vi "winchcontrol2014_preT-Tide.vi"() -> ()   [LabVIEW 2014]
uses:
  Instance           1 20Saved   winchcontrol .vi
  Instance           2 20Saved   winchcontrol .vi
  Instance           4 20Saved   winchcontrol .vi
  Instance           3 20Saved   winchcontrol .vi
  Instance           5 20Saved   winchcontrol .vi
  Instance           6 20Saved   winchcontrol .vi
panel:
  in  "Path of Image Capture":path=path "/OPG_Winch_MiniCoreDuo/Users/opg/Sites/FCTD_WINCH/LabView.png"
  in  "Screen Capture":bool
  out "Last update string":string="Updated: 10/29/12 6:37:41 PM"
  in  "Port":i32=4050
  in  "Red Lion IP Address":string="192.168.1.160"
  in  "Beep\non wait?":bool=TRUE
  in  "Drive by \nCTD Data":bool=TRUE
  out "isMaxPaySet":bool
  out "Old Max Payout":dbl=500.0
  in  "Maximum depth [m]":dbl=330.0 min=0.0 max=2000.0 step=1.0 format="%#_4f"
  out "Time @ max":timestamp=timestamp(3434357554.995505 s since 1904-01-01) format="%<%H:%M:%S>T"
  out "Max payout":dbl=26.1 format="%#_6f"
  out "Max depth":dbl format="%#_6f"
  in  "Go Up Now":bool
  in  "EMERGENCY\n      STOP":bool=TRUE caption="STOP!!!!!"
  in  "Final In Speed\n[turns/sec]":dbl=0.7 min=0.0 max=4.0 step=0.1 format="%_2f"
  in  "Slow depth\n[turns]":dbl=7.0 min=0.0 max=1500.0 step=1.0
  out "Final in Speed":dbl=0.7 min=0.0 max=4.0 step=0.1 format="%3_2g"
  out "Slow Depth":dbl=7.0 min=0.0 max=4.0 step=0.1
  out "Depth Derivative":dbl(graph)=0.09403073471738166
  out "CTD Com Miss Count":dbl
  out "Winch Com Miss Count":dbl=1.0
  out "Sax Status":u8[](array[numeric])=[1, 1, 0, 0, 5, 0, 1, 1, 0, 0]
  out "Pressure":dbl(graph)=1.818078
  out "i value":i32
  out "concatenated string":string="$OPGST,1,2,1243"
  out "CTD data":string="2615984408,1.818078,23.842880,5.097004"
  out "Depth":dbl(slide)=1.8080824462346528 min=0.0 max=1200.0 scale format="%#_4f"
  out "*(type *) &x":i32=38
  out "timestamp":u32=2615984408
  out "Temperature":dbl(graph)=23.84288
  out "Parameter String":string="$reqparmx:0019;0000$OPGWPM,10,16,+   6,+ 500, 4.2, 2.0,10000,10000,20000,40000,60000,60000,    0.70,    7,;"
  out "Status String":string="$OPGWST,3,1,+   1.8, 266.9,   0,- 0.01,   0.00,   0,   26307,;"
  out "Sax Status Code":dbl=26307.0 format="%#_8f"
  out "Motor Current":dbl
  out "Motor Payout":dbl=266.9
  out "Sheave Payout":dbl
  out "ATM90 Payout":dbl=1.8
  in  "CTD Data  IP Address":string="192.168.1.158"
  in  "Port":i32=2342
  out "bytes written":i32=62
  out "RL Status Received":bool=TRUE
  out "Acc Out":dbl=10000.0
  out "Acc In":dbl=10000.0
  out "Winch Action Status":T1(ring)=enum."HOMING"
  out "Winch Control Mode":T2(ring)=enum."AUTO"
  out "Decel Stop In":dbl=60000.0
  out "Decel Stop Out":dbl=60000.0
  out "Decel In":dbl=40000.0
  out "Decel Out":dbl=20000.0
  out "Wire In Speed":dbl=2.0
  out "Wire Out Speed":dbl=4.2
  out "Min Payout":dbl=6.0
  out "Max Payout":dbl=500.0
  out "I Limit Out":dbl=10.0
  out "I Limit In":dbl=16.0
  in  "Drop time [min.]":dbl=8.099999999999985 min=0.0 step=0.1 format="%.1f"
  out "output":string
  in  "Stop Now":bool
  in  "Wire In Speed\n[turns/sec]":dbl=2.0 min=0.0 max=5.0 step=0.1 format="%3_2f"
  in  "Decel in":dbl=40000.0
  in  "Decel out":dbl=20000.0
  in  "Stop decel in":dbl=60000.0
  in  "Stop decel out":dbl=60000.0
  in  "Accel  in":dbl=10000.0
  in  "Accel out":dbl=10000.0
  in  "Current limit out\n[Amps]":dbl=10.0 min=0.0 max=20.0 step=0.1 format="%_3f"
  in  "Current limit in\n[Amps]":dbl=16.0 min=0.0 max=18.0 format="%_3f"
  out "input 2":string="$reqparmx:0019;0000$OPGWPM,10,16,+   6,+ 500, 4.2, 2.0,10000,10000,20000,40000,60000,60000,    0.70,    7,;"
  out "Depth History":cluster{"Depth":dbl, "Value":dbl}(graph)={"Depth"=1.818078, "Value"=1.8}
  out "Payout":dbl(slide)=1.8 min=0.0 max=1200.0 step=200.0 scale format="%#1_3f"
  out "Velocity Now":dbl(knob)=-0.01 min=-5.0 max=5.0 step=1.0 scale=-5.0..5.0 scale format="%#_1f"
  in  "Maximum payout [turns]":dbl=500.0 min=0.0 max=1640.0 step=1.0 format="%#_4f"
  in  "Minimum payout [turns]":dbl=6.0 min=0.0 max=2000.0 step=1.0
  in  "Winch Auto Run":bool=TRUE
  out "Enabled":bool=TRUE
  in  "Wire Out Speed\n[turns/sec]":dbl=4.2 min=0.0 max=8.0 step=0.1 format="%_2f"
  out "Target\nDepth":dbl
  out "Conductivity":dbl(graph)=5.097004
  # "OPG  FAST  CTD"
  # "Winch Variable Status"
  # "Winch Variable Controls"
  # "FCTD DATA COMMUNICATION SETUP"
  # "RED LION CONTROL PANEL COM."
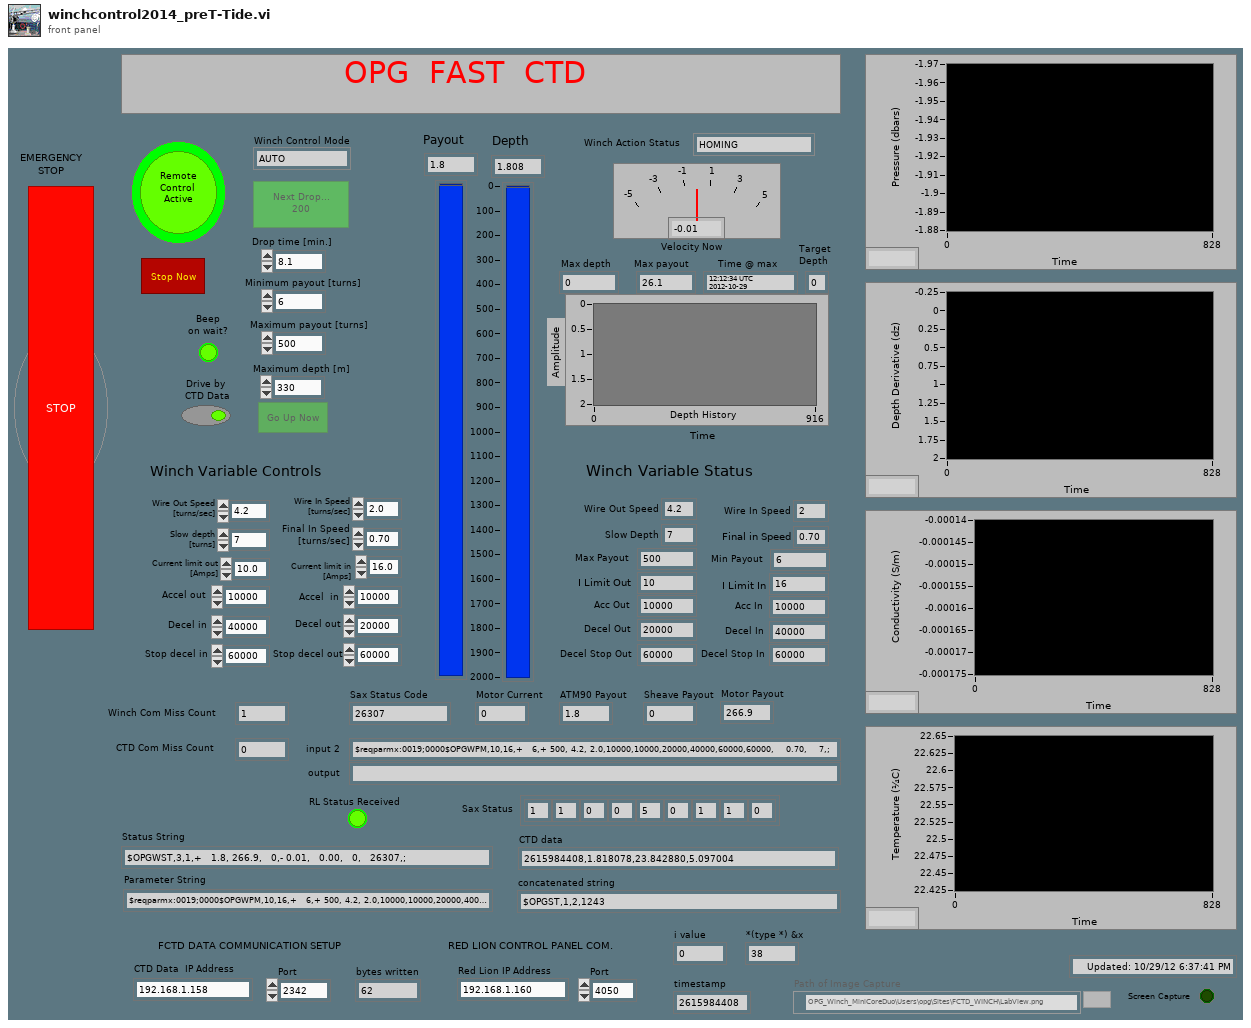
[diagram p1: front panel]
types:
  T1 = enum16{"START HOMING", "HOMING", "WAIT FOR TRIGGER", "START DROP", "GOING DOWN ?", "GOING UP"}
  T2 = enum16{"STOPPED", "MANUAL JOY", "MANUAL POT", "AUTO", "SEMIAUTO"}
  T3 = cluster{"Array[0]":dbl, "Array[1]":dbl, "Array[2]":dbl, "Array[3]":dbl, "Array[4]":dbl, "Array[5]":dbl, "Array[6]":dbl, "Array[7]":dbl, "Array[8]":dbl}
  T4 = cluster{"Array[0]":dbl, "Array[1]":dbl, "Array[2]":dbl, "Array[3]":dbl, "Array[4]":dbl, "Array[5]":dbl, "Array[6]":dbl, "Array[7]":dbl, "Array[8]":dbl, "Array[9]":dbl, "Array[10]":dbl, "Array[11]":dbl, "Array[12]":dbl, "Array[13]":dbl}
  T5 = typedef "imagedata.ctl" = cluster{"image type":i32, "image depth":i32, "image":u8[], "mask":u8[], "colors":u32[], "Rectangle":cluster{"left":i16, "top":i16, "right":i16, "bottom":i16}}
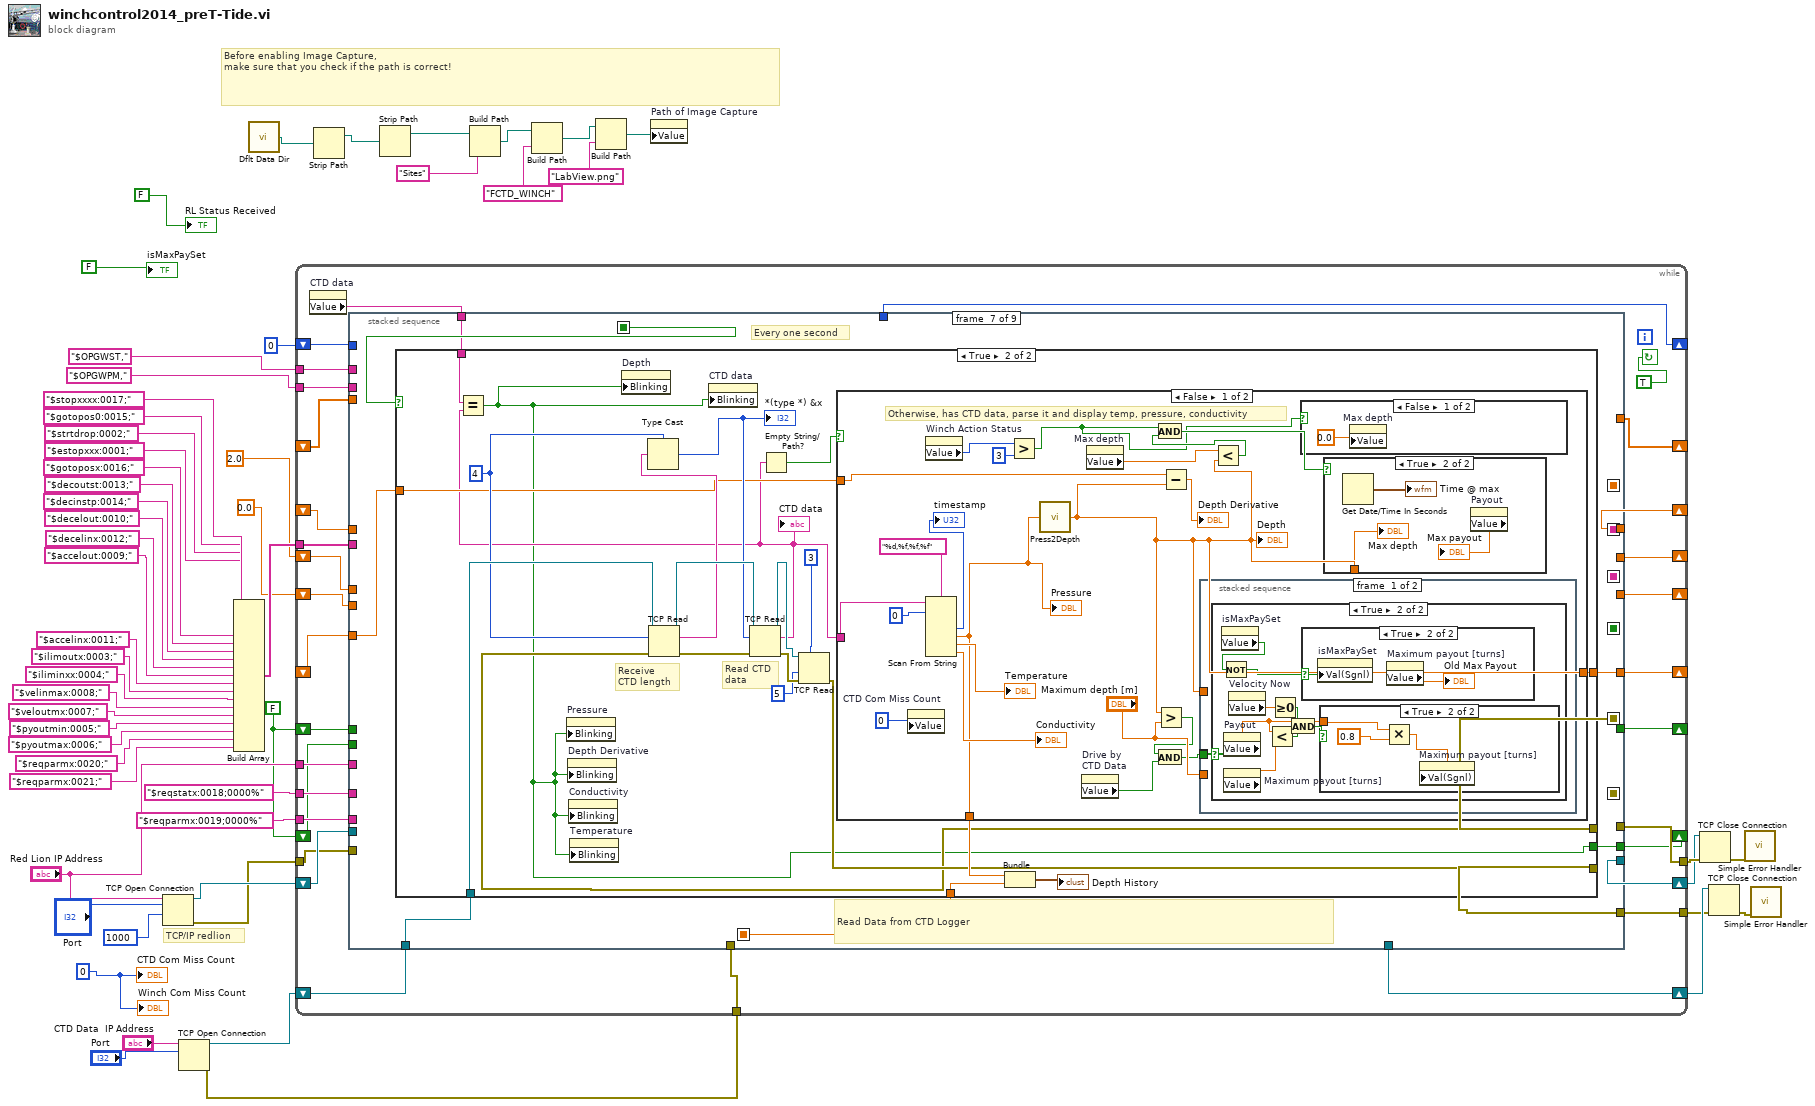
[diagram p0: block diagram]
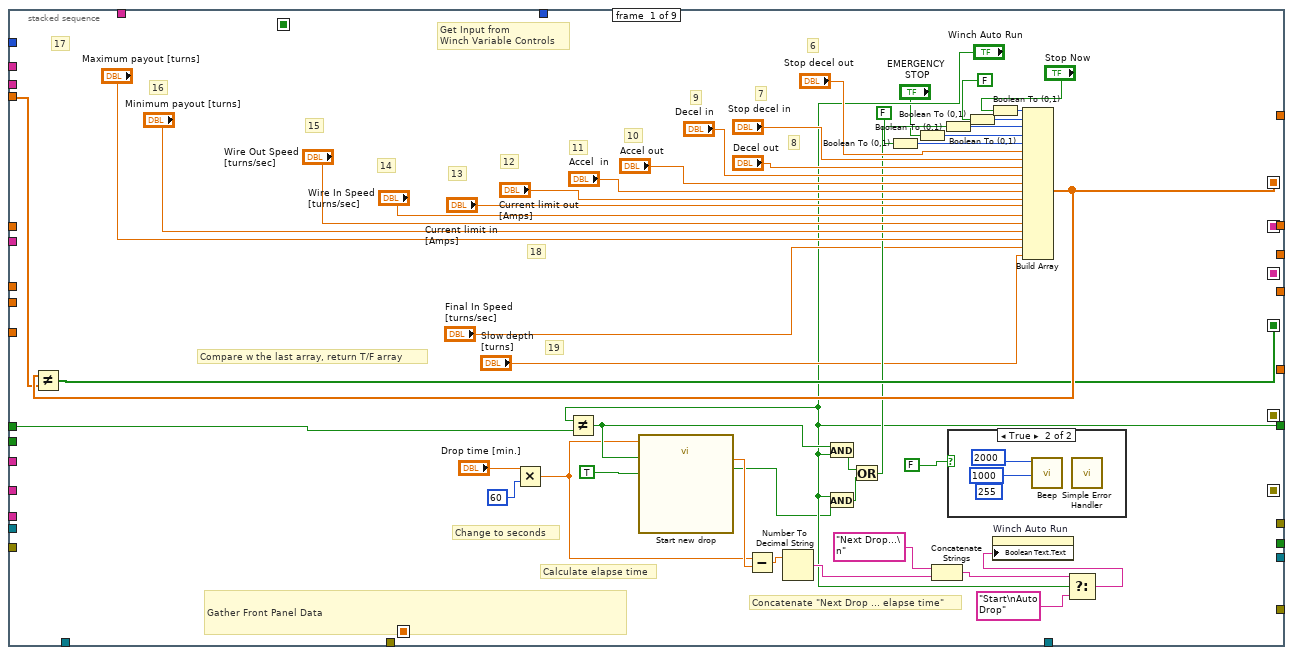
[diagram p2: hidden frame]
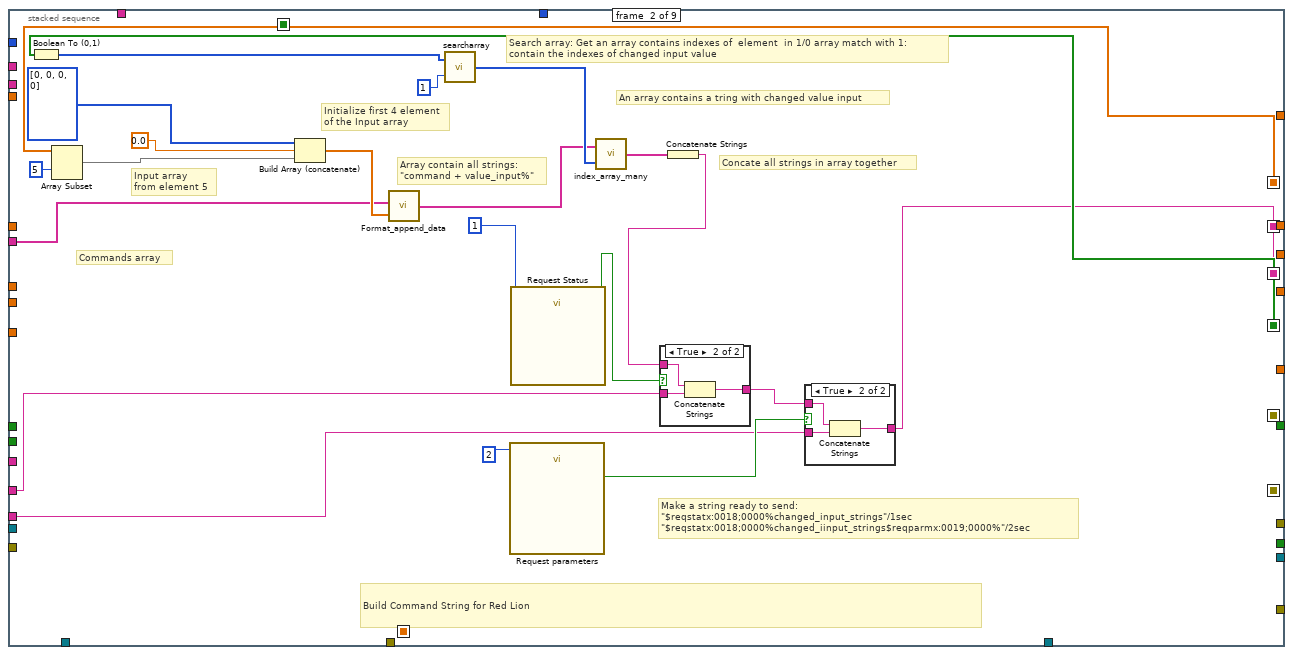
[diagram p4: hidden frame]
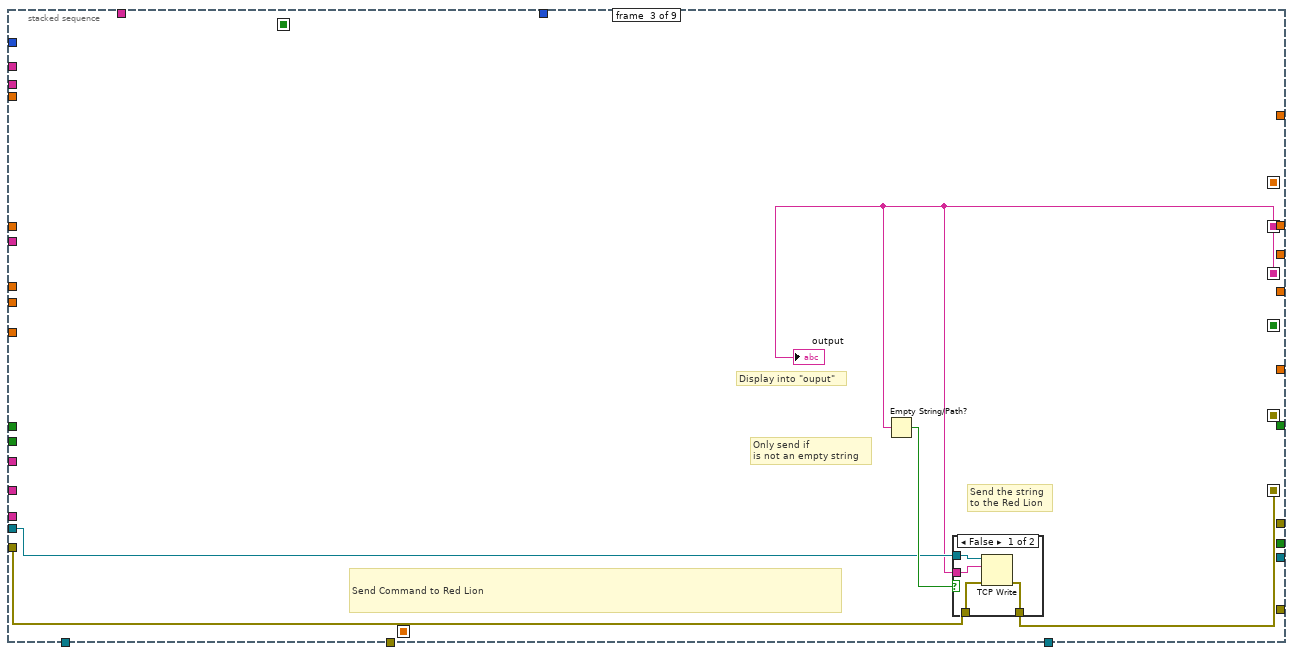
[diagram p7: hidden frame]
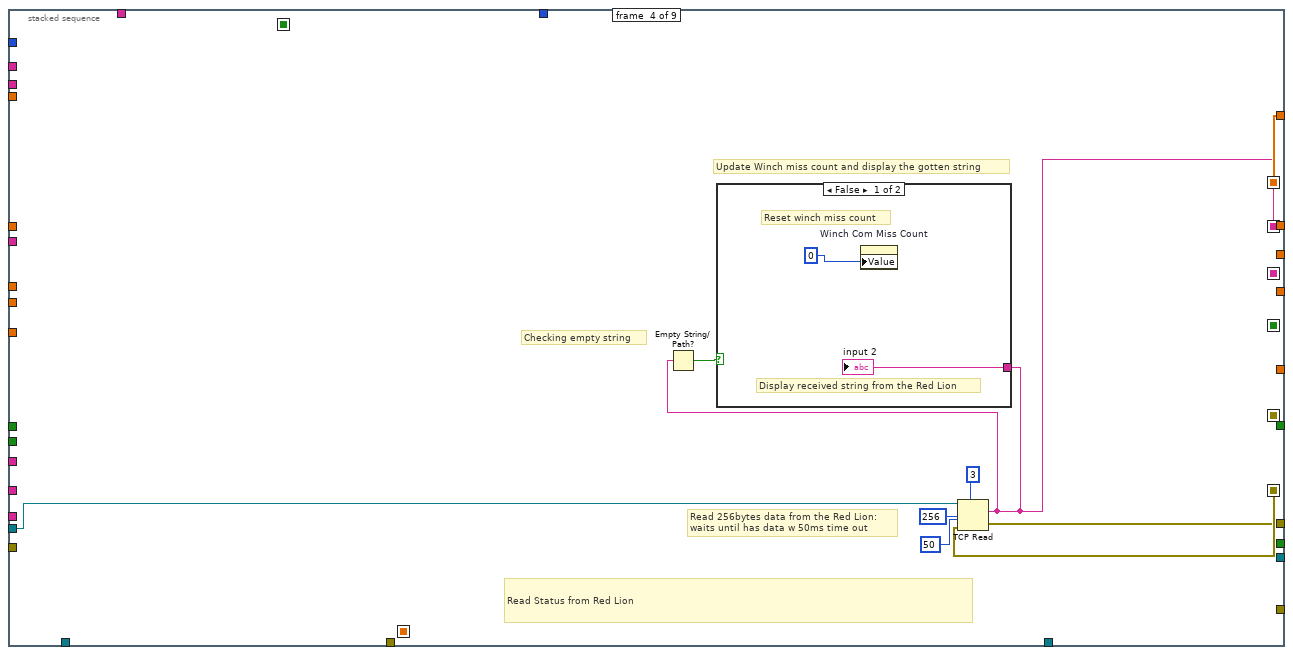
[diagram p9: hidden frame]
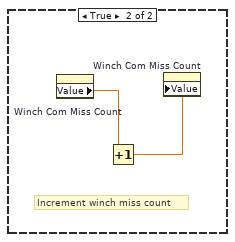
[diagram p10: hidden frame]
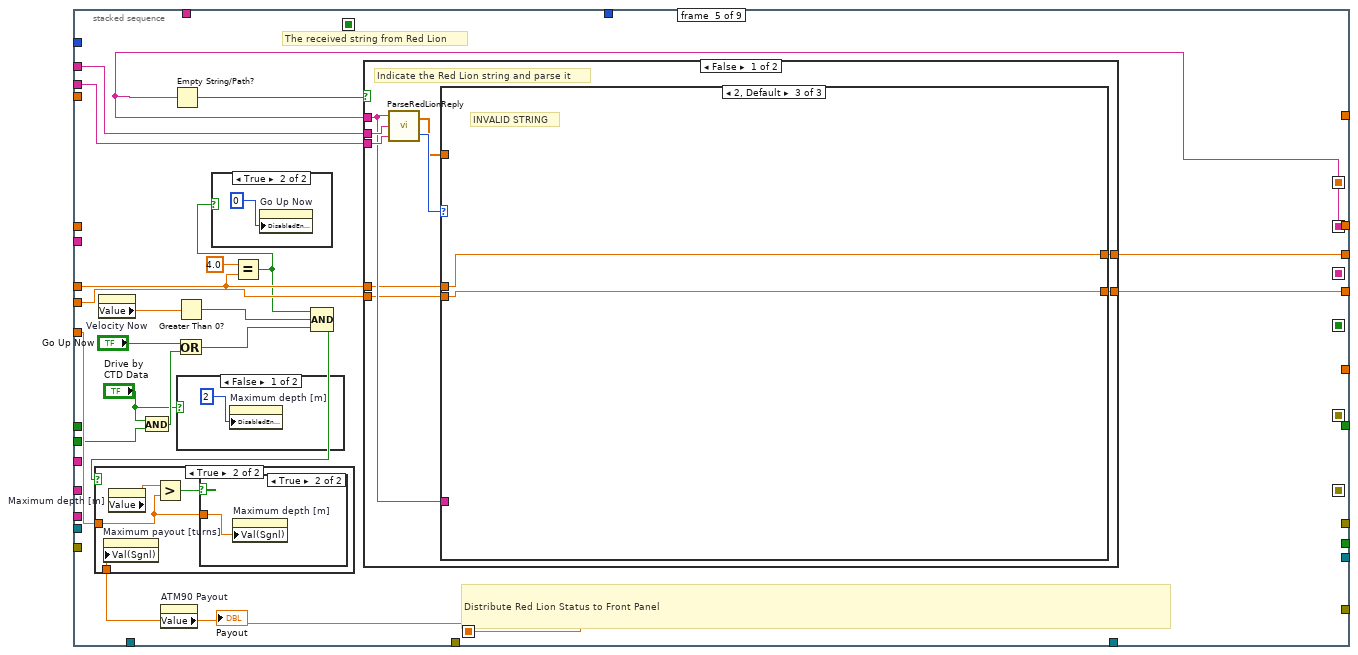
[diagram p11: hidden frame]
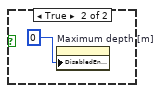
[diagram p12: hidden frame]
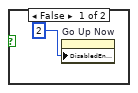
[diagram p13: hidden frame]
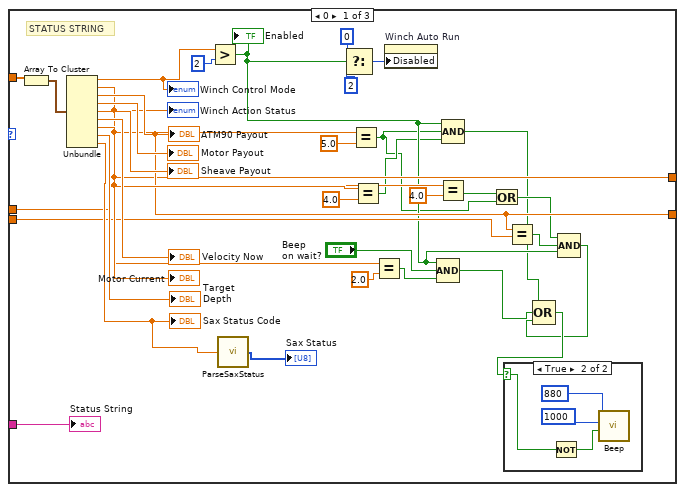
[diagram p16: hidden frame]
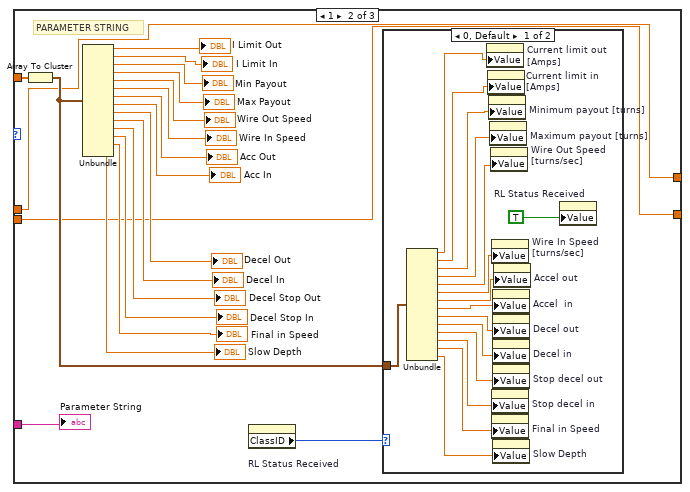
[diagram p18: hidden frame]
diagram:
  w12 = FALSE
  w19 = 0
  # "Before enabling Image Capture, \nmake sure that you check if the path is correct!"
  # "TCP/IP redlion"
  n1 = TCP Open Connection(address="Red Lion IP Address", remote port or service name="Port", timeout ms (60000)=1000) -> (connection ID=w54:refnum<k5>, error out=w52:errorcluster)  [unwired: 2 in]
  n2 = TCP Open Connection(address="CTD Data  IP Address", remote port or service name="Port") -> (connection ID=w28:refnum<k5>, error out=w26:errorcluster)  [unwired: 3 in]
  n3 = Build Array("$stopxxxx:0017;", "$gotopos0:0015;", "$strtdrop:0002;", "$estopxxx:0001;", "$gotoposx:0016;", "$decoutst:0013;", "$decinstp:0014;", "$decelout:0010;", "$decelinx:0012;", "$accelout:0009;", "$accelinx:0011;", "$ilimoutx:0003;", "$iliminxx:0004;", "$velinmax:0008;", "$veloutmx:0007;", "$pyoutmin:0005;", "$pyoutmax:0006;", "$reqparmx:0020;", "$reqparmx:0021;") -> (w50:string[])
  n4 = call <vilib>:"Dflt Data Dir.vi"() -> ("App:Default Data Directory"=w9:path)
  n5 = while {
    shift-right: [w87] -> _
    shift-left: _ -> [w85]
    tunnel: w52 -> [w82]
    tunnel: [w86] -> w51
    tunnel: w50 -> [w84]
    tunnel: "$reqstatx:0018;0000%" -> [w81]
    shift-right: [w80] -> _
    shift-left: w12 -> [w79]
    tunnel: w26 -> [w77]
    tunnel: [w76] -> w25
    tunnel: "$reqparmx:0019;0000%" -> [w75]
    shift-right: [w74] -> _
    shift-left: _ -> [w73]
    shift-right: [w72] -> _
    shift-left: 0 -> [w71]
    tunnel: "$OPGWST," -> [w70]
    tunnel: "$OPGWPM," -> [w69]
    shift-right: [w67] -> w18
    shift-left: w54 -> [w83]
    shift-right: [w66] -> w27
    shift-left: w28 -> [w78]
    shift-right: [w65] -> _
    shift-left: _ -> [w64]
    tunnel: "Red Lion IP Address" -> [w62]
    shift-right: [w61] -> _
    shift-left: w12 -> [w60]
    shift-right: [w59] -> _
    shift-left: 2.0 -> [w58]
    shift-right: [w57] -> _
    shift-left: 0.0 -> [w56]
    stop <- TRUE continue-if-true
    n6 = property on="CTD data" class="Str"() -> ("Value"=w63:string)  [unwired: 2 in, 2 out]
    n7 = stacked-sequence {
      seq-local: [w132 _ _ _ _ _ _ _ _] -> [_ w149 _ w183 _ _ _ _ _]
      seq-local: [_ w135 _ _ _ _ _ _ _] -> [_ _ w165 _ _ _ _ _ _]
      seq-local: [_ _ w166 _ _ _ _ _ _] -> [_ _ _ w178 _ _ _ _ _]
      seq-local: [w128 _ _ _ _ _ _ _ _] -> [_ w156 _ _ _ _ _ _ _]
      seq-local: [_ _ _ w176 _ _ _ _ _] -> [_ _ _ _ w205 _ _ _ _]
      seq-local: [_ _ _ _ _ w311 _ _ _] -> [_ _ _ _ _ _ w357 _ _]
      seq-local: [_ _ _ _ w203 _ _ _ _] -> [_ _ _ _ _ _ w355 _ _]
      seq-local: [_ _ _ _ _ w310 _ _ _] -> [_ _ _ _ _ _ w354 _ _]
      tunnel: w82 -> [_ _ w168 _ _ _ _ _ _]
      tunnel: w83 -> [_ _ w167 w179 _ _ _ w445 _]
      tunnel: [_ _ _ w183 _ _ _ _ _] -> w87
      tunnel: w84 -> [_ w147 _ _ _ _ _ _ _]
      tunnel: [_ _ _ w177 _ _ _ _ _] -> w86
      tunnel: w85 -> [w131 _ _ _ _ _ _ _ _]
      tunnel: w81 -> [_ w141 _ _ _ _ _ _ _]
      tunnel: ["Winch Auto Run" _ _ _ _ _ _ _ _] -> w80
      tunnel: w79 -> [w106 _ _ _ _ _ _ _ _]
      tunnel: w78 -> [_ _ _ _ _ w313 w358 w443 _]
      tunnel: w77 -> [_ _ _ _ _ w312 _ _ _]
      tunnel: [_ _ _ _ _ _ w356 _ _] -> w76
      tunnel: w75 -> [_ w136 _ _ _ _ _ _ _]
      tunnel: [_ _ _ _ _ w308 _ _ _] -> w74
      tunnel: w73 -> [_ _ _ _ _ w307 _ _ _]
      tunnel: w71 -> [_ _ _ _ _ w306 _ _ _]
      tunnel: [_ _ _ _ _ w305 _ _ _] -> w72
      tunnel: w70 -> [_ _ _ _ w207 _ _ _ _]
      tunnel: w69 -> [_ _ _ _ w206 _ _ _ _]
      tunnel: [_ _ _ _ _ _ _ w444 _] -> w67
      tunnel: [_ _ _ _ _ _ _ w442 _] -> w66
      tunnel: [_ _ _ _ _ _ w353 _ _] -> w65
      tunnel: w64 -> [_ _ _ _ w199 _ w352 _ _]
      tunnel: w63 -> [_ _ _ _ _ _ w351 _ _]
      tunnel: w62 -> [_ _ _ _ _ _ _ w441 _]
      tunnel: [_ _ _ _ _ _ w350 _ _] -> w61
      tunnel: w60 -> [_ _ _ _ w196 _ _ _ _]
      tunnel: [_ _ _ _ w193 _ _ _ _] -> w59
      tunnel: w58 -> [_ _ _ _ w189 _ _ _ _]
      tunnel: [_ _ _ _ w192 _ _ _ _] -> w57
      tunnel: w56 -> [_ _ _ _ w191 _ _ _ _]
      frame #0 {
        w129 = FALSE items=["OFF", "ON", "OFF", "ON"] ("Return to top")
        w115 = FALSE items=["OFF", "ON", "OFF", "ON"] ("Go to ...")
        # "19"
        # "18"
        # "17"
        # "16"
        # "15"
        # "14"
        # "13"
        # "12"
        # "11"
        # "10"
        # "9"
        # "8"
        # "7"
        # "6"
        # "Compare w the last array, return T/F array"
        # "Concatenate \"Next Drop ... elapse time\""
        # "Calculate elapse time"
        # "Change to seconds"
        # "Get Input from\nWinch Variable Controls"
        # "Gather Front Panel Data"
        n8 = Multiply(x="Drop time [min.]", y=60) -> (x*y=w100:dbl)
        n9 = Not Equal?(x="Winch Auto Run", y=w106) -> (x != y?=w105:bool)
        n10 = call "Start new drop"("Time Target (s)"=w100, "Reset"=w105, "Auto Reset"=TRUE) -> ("Elapsed Time (s)"=w101:dbl, "Time has Elapsed"=w90:bool)  [unwired: 9 in, 6 out]
        n11 = Subtract(x=w100, y=w101) -> (x-y=w99:dbl)
        n12 = Number To Decimal String(number=w99) -> (decimal integer string=w98:string)  [unwired: 1 in]
        n13 = And(x=w105, y="Winch Auto Run") -> (x .and. y?=w104:bool)
        n14 = And(x="Winch Auto Run", y=w90) -> (x .and. y?=w103:bool)
        n15 = Or(x=w104, y=w103) -> (x .or. y?=w102:bool)
        n16 = Boolean To (0,1)(Boolean=w115) -> (0, 1=w114:i16)
        n17 = Boolean To (0,1)(Boolean="EMERGENCY\n      STOP") -> (0, 1=w113:i16)
        n18 = Concatenate Strings("Next Drop...\n", w98) -> (w95:string)
        n19 = Boolean To (0,1)(Boolean=w102) -> (0, 1=w112:i16)
        n20 = case shown="True" FALSE {
          frame False {
          }
          frame True {
            (unwired) 255
            n21 = call <vilib>:"Beep.vi"("duration (msec) - ignored"=1000, "frequency (Hz) - ignored"=2000) -> ()  [unwired: 10 in]
            n22 = call <vilib>:"Simple Error Handler.vi"() -> ()  [unwired: 5 in, 5 out]
          }
        }
        n23 = Boolean To (0,1)(Boolean=w129) -> (0, 1=w111:i16)
        n24 = Boolean To (0,1)(Boolean="Stop Now") -> (0, 1=w110:i16)
        n25 = Build Array(w110, w111, w112, w113, w114, "Stop decel out", "Stop decel in", "Decel out", "Decel in", "Accel out", "Accel  in", "Current limit out\n[Amps]", "Current limit in\n[Amps]", "Wire In Speed\n[turns/sec]", "Wire Out Speed\n[turns/sec]", "Minimum payout [turns]", "Maximum payout [turns]", "Final In Speed\n[turns/sec]", "Slow depth\n[turns]") -> (w132:dbl[])
        n26 = Not Equal?(x=w132, y=w131) -> (x != y?=w128:bool[])
        n27 = Select(t=w95, s="Winch Auto Run", f="Start\nAuto Drop") -> (s? t:f=w96:string)
        n28 = property on="Winch Auto Run" class="Bool (strict)"("Boolean Text.Text"=w96) -> ()  [unwired: 2 in, 2 out]
      }
      frame #1 {
        # "Make a string ready to send:\n\"$reqstatx:0018;0000%changed_input_strings\"/1sec\n\"$reqstatx:0018;0000%changed_iinput_strings$reqparmx:0019;0000%\"/2sec"
        # "Concate all strings in array together"
        # "An array contains a tring with changed value input"
        # "Array contain all strings:\n\"command + value_input%\""
        # "Commands array"
        # "Initialize first 4 element\nof the Input array"
        # "Input array\nfrom element 5"
        # "Search array: Get an array contains indexes of  element  in 1/0 array match with 1:\ncontain the indexes of changed input value"
        # "Build Command String for Red Lion"
        n29 = Boolean To (0,1)(Boolean=w156) -> (0, 1=w154:i16[])
        n30 = Array Subset(array=w149, index=5) -> (w145:dbl[])  [unwired: 1 in]
        n31 = Build Array (concatenate)(i32[] [0, 0, 0, 0], 0.0 ("Depth to go to"), w145) -> (w148:dbl[])
        n32 = call "Format_append_data.vi"("Numbers to append"=w148, "Strings without numbers"=w147) -> ("Final Strings"=w146:string[])
        n33 = call "searcharray.vi"("Search character"=1, "Array 2"=w154) -> ("Array"=w153:i16[])
        n34 = call "Request parameters"("Time Target (s)"=2) -> ("Time has Elapsed"=w137:bool)  [unwired: 11 in, 7 out]
        n35 = call "Request Status"("Time Target (s)"=1) -> ("Time has Elapsed"=w142:bool)  [unwired: 11 in, 7 out]
        n36 = call "index_array_many.vi"("Lines of Array to grab"=w153, "String Array Input"=w146) -> ("Output array"=w152:string[])
        n37 = Concatenate Strings(w152) -> (w140:string)
        n38 = case shown="True" w142 {
          tunnel: w140 -> [w161 w164]
          tunnel: [w161 w163] -> w138
          tunnel: w141 -> [_ w162]
          frame False {
          }
          frame True {
            n39 = Concatenate Strings(w164, w162) -> (w163:string)
          }
        }
        n40 = case shown="True" w137 {
          tunnel: w138 -> [w157 w160]
          tunnel: [w157 w159] -> w135
          tunnel: w136 -> [_ w158]
          frame False {
          }
          frame True {
            n41 = Concatenate Strings(w160, w158) -> (w159:string)
          }
        }
      }
      frame #2 {
        # "Send the string\nto the Red Lion"
        # "Only send if\nis not an empty string"
        # "Display into \"ouput\""
        # "Send Command to Red Lion"
        n42 = Empty String/Path?(string/path=w165) -> (empty?=w169:bool)
        n43 = case shown="False" w169 {
          tunnel: w165 -> [w172 _]
          tunnel: w167 -> [w173 _]
          tunnel: w168 -> [w171 w174]
          tunnel: [w170 w174] -> w166
          frame False {
            n44 = TCP Write(connection ID=w173, data in=w172, error in (no error)=w171) -> (error out=w170:errorcluster)  [unwired: 1 in, 2 out]
          }
          frame True {
          }
        }
        "output" <- w165
      }
      frame #3 {
        # "Update Winch miss count and display the gotten string"
        # "Checking empty string"
        # "Read 256bytes data from the Red Lion:\nwaits until has data w 50ms time out"
        # "Read Status from Red Lion"
        n45 = TCP Read(connection ID=w179, bytes to read=256, error in (no error)=w178, 7:3, 9:50) -> (data out=w176:string, error out=w177:errorcluster)  [unwired: 1 out]
        n46 = Empty String/Path?(string/path=w176) -> (empty?=w175:bool)
        n47 = case shown="False" w175 {
          tunnel: w176 -> [w185 _]
          frame False {
            # "Display received string from the Red Lion"
            # "Reset winch miss count"
            n48 = property on="Winch Com Miss Count" class="DigNum (strict)"("Value"=0) -> ()  [unwired: 2 in, 2 out]
            "input 2" <- w185
          }
          frame True {
            # "Increment winch miss count"
            n49 = property on="Winch Com Miss Count" class="DigNum (strict)"() -> ("Value"=w187:dbl)  [unwired: 2 in, 2 out]
            n50 = Increment(x=w187) -> (x+1=w186:dbl)
            n51 = property on="Winch Com Miss Count" class="DigNum (strict)"("Value"=w186) -> ()  [unwired: 2 in, 2 out]
          }
        }
      }
      frame #4 {
        # "The received string from Red Lion"
        # "Distribute Red Lion Status to Front Panel"
        n52 = property on="Velocity Now" class="Knob (strict)"() -> ("Value"=w202:dbl)  [unwired: 2 in, 2 out]
        n53 = And(x="Drive by \nCTD Data", y=w196) -> (x .and. y?=w195:bool)
        n54 = property on="ATM90 Payout" class="DigNum (strict)"() -> ("Value"=w203:dbl)  [unwired: 2 in, 2 out]
        "Payout" <- w203
        n55 = Empty String/Path?(string/path=w205) -> (empty?=w204:bool)
        n56 = Greater Than 0?(x=w202) -> (x > 0?=w200:bool)
        n57 = Or(x="Go Up Now", y=w195) -> (x .or. y?=w197:bool)
        n58 = case shown="False" "Drive by \nCTD Data" {
          frame False {
            n59 = property on="Maximum depth [m]" class="DigNum (strict)"("DisabledEnum"=2) -> ()  [unwired: 2 in, 2 out]
          }
          frame True {
            n60 = property on="Maximum depth [m]" class="DigNum (strict)"("DisabledEnum"=0) -> ()  [unwired: 2 in, 2 out]
          }
        }
        n61 = Equal?(x=4.0, y=w189) -> (x = y?=w188:bool)
        n62 = case shown="True" w188 {
          frame False {
            n63 = property on="Go Up Now" class="Bool"("DisabledEnum"=2) -> ()  [unwired: 2 in, 2 out]
          }
          frame True {
            n64 = property on="Go Up Now" class="Bool"("DisabledEnum"=0) -> ()  [unwired: 2 in, 2 out]
          }
        }
        n65 = Compound Arithmetic op=AND(w188, w200, w197) -> (w201:bool)
        n66 = case shown="True" w201 {
          tunnel: w203 -> [_ w215]
          tunnel: w199 -> [_ w212]
          frame False {
          }
          frame True {
            n67 = property on="Maximum payout [turns]" class="DigNum (strict)"("Val(Sgnl)"=w215) -> ()  [unwired: 2 in, 2 out]
            n68 = property on="Maximum depth [m]" class="DigNum (strict)"() -> ("Value"=w214:dbl)  [unwired: 2 in, 2 out]
            n69 = Greater?(x=w214, y=w212) -> (0:w213:bool)
            n70 = case shown="True" w213 {
              tunnel: w212 -> [_ w216]
              frame False {
              }
              frame True {
                n71 = property on="Maximum depth [m]" class="DigNum (strict)"("Val(Sgnl)"=w216) -> ()  [unwired: 2 in, 2 out]
              }
            }
          }
        }
        n72 = case shown="False" w204 {
          tunnel: w207 -> [w223 _]
          tunnel: w206 -> [w222 _]
          tunnel: w205 -> [w221 _]
          tunnel: [w220 w304] -> w193
          tunnel: w189 -> [w219 w304]
          tunnel: [w218 w303] -> w192
          tunnel: w191 -> [w217 w303]
          frame False {
            # "Indicate the Red Lion string and parse it"
            n73 = call "ParseRedLionReply.vi"("Parameter Iidicator"=w222, "Status Indicator"=w223, "Red Lion String"=w221) -> ("Type"=w225:i16, "Array"=w224:dbl[])
            n74 = case shown="2, Default" w225 {
              tunnel: w224 -> [w259 w284 _]
              tunnel: w221 -> [w251 w270 _]
              tunnel: [w238 w267 w302] -> w220
              tunnel: w219 -> [w242 w267 w302]
              tunnel: [w241 w266 w301] -> w218
              tunnel: w217 -> [w240 w266 w301]
              frame 0 {
                # "STATUS STRING"
                n75 = Array To Cluster(array=w259) -> (cluster=w258:T3)
                n76 = Unbundle(w258) -> ("Array[0]"=w257:dbl, "Array[1]"=w238:dbl, "Array[2]"=w241:dbl, "Array[3]"=→"Motor Payout":dbl, "Array[4]"=→"Sheave Payout":dbl, "Array[5]"=→"Velocity Now":dbl, "Array[6]"=→"Motor Current":dbl, "Array[7]"=→"Target\nDepth":dbl, "Array[8]"=w247:dbl)
                "Winch Control Mode" <- w257
                "Winch Action Status" <- w238
                "ATM90 Payout" <- w241
                "Sax Status Code" <- w247
                n77 = Greater?(x=w257, y=2) -> (0:w234:bool)
                "Enabled" <- w234
                n78 = call "ParseSaxStatus.vi"("Status Code In"=w247) -> ("Status Flags"=→"Sax Status":i8[])
                n79 = Select(t=0, s=w234, f=2) -> (s? t:f=w248:i32)
                n80 = Equal?(x=w238, y=5.0) -> (x = y?=w227:bool)
                n81 = Equal?(x=w242, y=4.0) -> (x = y?=w231:bool)
                n82 = Equal?(x=w238, y=2.0) -> (x = y?=w233:bool)
                n83 = property on="Winch Auto Run" class="Bool (strict)"("Disabled"=w248) -> ()  [unwired: 2 in, 2 out]
                n84 = Compound Arithmetic op=AND(w234, "Beep\non wait?", w233) -> (w228:bool)
                n85 = Equal?(x=w238, y=4.0) -> (x = y?=w237:bool)
                n86 = Compound Arithmetic op=AND(w234, w227, w231) -> (w230:bool)
                n87 = Or(x=w237, y=w227) -> (x .or. y?=w236:bool)
                n88 = Equal?(x=w241, y=w240) -> (x = y?=w235:bool)
                n89 = Compound Arithmetic op=AND(w236, w235, w234) -> (w226:bool)
                n90 = Compound Arithmetic op=OR(w230, w228, w226) -> (w229:bool)
                n91 = case shown="True" w229 {
                  selector: w229 -> [_ w261]
                  frame False {
                  }
                  frame True {
                    n92 = Not(x=w261) -> (.not. x?=w262:bool)
                    n93 = call <vilib>:"Beep.vi"("use system alert? (T) - ignored"=w262, "duration (msec) - ignored"=u32 1000, "frequency (Hz) - ignored"=u32 880) -> ()  [unwired: 9 in]
                  }
                }
                "Status String" <- w251
              }
              frame 1 {
                # "PARAMETER STRING"
                n94 = Array To Cluster(array=w284) -> (cluster=w271:T4)
                n95 = Unbundle(w271) -> ("Array[0]"=→"I Limit Out":dbl, "Array[1]"=→"I Limit In":dbl, "Array[2]"=→"Min Payout":dbl, "Array[3]"=→"Max Payout":dbl, "Array[4]"=→"Wire Out Speed":dbl, "Array[5]"=→"Wire In Speed":dbl, "Array[6]"=→"Acc Out":dbl, "Array[7]"=→"Acc In":dbl, "Array[8]"=→"Decel Out":dbl, "Array[9]"=→"Decel In":dbl, "Array[10]"=→"Decel Stop Out":dbl, "Array[11]"=→"Decel Stop In":dbl, "Array[12]"=→"Final in Speed":dbl, "Array[13]"=→"Slow Depth":dbl)
                n96 = property on="RL Status Received" class="Bool (strict)"() -> ("ClassID"=w265:u32)  [unwired: 2 in, 2 out]
                n97 = case shown="0, Default" w265 {
                  tunnel: w271 -> [w300 _]
                  frame 0, Default {
                    n98 = Unbundle(w300) -> ("Array[0]"=w299:dbl, "Array[1]"=w298:dbl, "Array[2]"=w297:dbl, "Array[3]"=w296:dbl, "Array[4]"=w295:dbl, "Array[5]"=w294:dbl, "Array[6]"=w288:dbl, "Array[7]"=w293:dbl, "Array[8]"=w292:dbl, "Array[9]"=w291:dbl, "Array[10]"=w290:dbl, "Array[11]"=w289:dbl, "Array[12]"=w287:dbl, "Array[13]"=w286:dbl)
                    n99 = property on="Current limit out\n[Amps]" class="DigNum (strict)"("Value"=w299) -> ()  [unwired: 2 in, 2 out]
                    n100 = property on="Current limit in\n[Amps]" class="DigNum (strict)"("Value"=w298) -> ()  [unwired: 2 in, 2 out]
                    n101 = property on="Minimum payout [turns]" class="DigNum (strict)"("Value"=w297) -> ()  [unwired: 2 in, 2 out]
                    n102 = property on="Maximum payout [turns]" class="DigNum (strict)"("Value"=w296) -> ()  [unwired: 2 in, 2 out]
                    n103 = property on="Wire Out Speed\n[turns/sec]" class="DigNum (strict)"("Value"=w295) -> ()  [unwired: 2 in, 2 out]
                    n104 = property on="Wire In Speed\n[turns/sec]" class="DigNum (strict)"("Value"=w294) -> ()  [unwired: 2 in, 2 out]
                    n105 = property on="Stop decel in" class="DigNum (strict)"("Value"=w289) -> ()  [unwired: 2 in, 2 out]
                    n106 = property on="Final in Speed" class="DigNum (strict)"("Value"=w287) -> ()  [unwired: 2 in, 2 out]
                    n107 = property on="Accel  in" class="DigNum (strict)"("Value"=w293) -> ()  [unwired: 2 in, 2 out]
                    n108 = property on="Decel out" class="DigNum (strict)"("Value"=w292) -> ()  [unwired: 2 in, 2 out]
                    n109 = property on="Decel in" class="DigNum (strict)"("Value"=w291) -> ()  [unwired: 2 in, 2 out]
                    n110 = property on="Stop decel out" class="DigNum (strict)"("Value"=w290) -> ()  [unwired: 2 in, 2 out]
                    n111 = property on="Slow Depth" class="DigNum (strict)"("Value"=w286) -> ()  [unwired: 2 in, 2 out]
                    n112 = property on="Accel out" class="DigNum (strict)"("Value"=w288) -> ()  [unwired: 2 in, 2 out]
                    n113 = property on="RL Status Received" class="Bool (strict)"("Value"=TRUE) -> ()  [unwired: 2 in, 2 out]
                  }
                  frame 1 {
                  }
                }
                "Parameter String" <- w270
              }
              frame 2, Default {
                # "INVALID STRING"
              }
            }
          }
          frame True {
            # "If empty string, do nothing"
          }
        }
      }
      frame #5 {
        # "Send Status to CTD Logger"
        n114 = call "Send to FastCTD  logger"("Time Target (s)"=1) -> ("Time has Elapsed"=w310:bool)  [unwired: 11 in, 7 out]
        n115 = case shown="True" w310 {
          tunnel: w313 -> [_ w326]
          tunnel: w312 -> [w316 w325]
          tunnel: [w316 w324] -> w311
          tunnel: [w315 w320] -> w308
          tunnel: w307 -> [w315 w319]
          tunnel: w306 -> [w314 w318]
          tunnel: [w314 w317] -> w305
          frame False {
          }
          frame True {
            n116 = property on="Status String" class="Str"() -> ("Value"=w322:string)  [unwired: 2 in, 2 out]
            n117 = Empty String/Path?(string/path=w322) -> (empty?=w323:bool)
            n118 = case shown="True" w323 {
              tunnel: w322 -> [w330 _]
              tunnel: [w330 w340] -> w321
              tunnel: [w329 w334] -> w320
              tunnel: w319 -> [w329 w333]
              tunnel: w318 -> [w328 w332]
              tunnel: [w328 w331] -> w317
              frame False {
              }
              frame True {
                # "Since Status string is empty, make a string \"$OPGST,1,2/3,1243\"\nto send to FCTD app"
                n119 = Increment(x=w332) -> (x+1=w331:i32)
                n120 = Quotient & Remainder(x=w331, y=4) -> (x-y*floor(x/y)=w337:i32)  [unwired: 1 out]
                n121 = Equal To 0?(x=w337) -> (x = 0?=w336:bool)
                n122 = case shown="False" w336 {
                  tunnel: [w343 w345] -> w335
                  tunnel: [w343 w345] -> w334
                  tunnel: w333 -> [w343 w344]
                  frame False {
                  }
                  frame True {
                    n123 = Equal?(x=w344, y=3.0) -> (x = y?=w346:bool)
                    n124 = Select(t=2.0 ("y"), s=w346, f=3.0 ("y")) -> (s? t:f=w345:dbl)
                  }
                }
                n125 = Number To Decimal String(number=w335) -> (decimal integer string=w339:string)  [unwired: 1 in]
                n126 = Concatenate Strings("$OPGST,1," ("string"), w339, ",1243" ("string")) -> (w340:string)
                "concatenated string" <- w340
              }
            }
            n127 = TCP Write(connection ID=w326, data in=w321, error in (no error)=w325) -> (bytes written=→"bytes written":i32, error out=w324:errorcluster)  [unwired: 1 in, 1 out]
          }
        }
        "i value" <- w306
      }
      frame #6 {
        # "Every one second"
        # "Read Data from CTD Logger"
        n128 = case shown="True" w354 {
          selector: w354 -> [w359 _]
          tunnel: w358 -> [_ w382]
          tunnel: w357 -> [w361 w363]
          tunnel: [w361 w371] -> w356
          tunnel: w355 -> [_ w381]
          tunnel: [w360 w367] -> w353
          tunnel: w352 -> [w360 w366]
          tunnel: w351 -> [_ w364]
          tunnel: [w359 w362] -> w350
          frame False {
          }
          frame True {
            w380 = 4
            # "Read CTD\ndata"
            # "Receive\nCTD length"
            n129 = TCP Read(connection ID=w382, bytes to read=w380, error in (no error)=w363) -> (connection ID out=w379:refnum<k5>, data out=w378:string, error out=w376:errorcluster)  [unwired: 2 in]
            n130 = Type Cast(type=w380, x=w378) -> (*(type *) &x=w377:i32)
            "*(type *) &x" <- w377
            n131 = TCP Read(connection ID=w379, bytes to read=w377, error in (no error)=w376) -> (connection ID out=w370:refnum<k5>, data out=w365:string, error out=w372:errorcluster)  [unwired: 2 in]
            "CTD data" <- w365
            n132 = Equal?(x=w364, y=w365) -> (x = y?=w362:bool)
            n133 = property on="Pressure" class="WFChart (strict)"("Blinking"=w362) -> ()  [unwired: 2 in, 2 out]
            n134 = property on="Depth Derivative" class="WFChart (strict)"("Blinking"=w362) -> ()  [unwired: 2 in, 2 out]
            n135 = property on="Conductivity" class="WFChart (strict)"("Blinking"=w362) -> ()  [unwired: 2 in, 2 out]
            n136 = property on="Temperature" class="WFChart (strict)"("Blinking"=w362) -> ()  [unwired: 2 in, 2 out]
            n137 = property on="Depth" class="Slide (strict)"("Blinking"=w362) -> ()  [unwired: 2 in, 2 out]
            n138 = property on="CTD data" class="Str"("Blinking"=w362) -> ()  [unwired: 2 in, 2 out]
            n139 = Empty String/Path?(string/path=w365) -> (empty?=w374:bool)
            n140 = TCP Read(connection ID=w370, error in (no error)=w372, 7:3, 9:5) -> (error out=w371:errorcluster)  [unwired: 1 in, 2 out]
            n141 = case shown="False" w374 {
              tunnel: w365 -> [w396 _]
              tunnel: [w390 0.0] -> w375
              tunnel: [w387 w438] -> w367
              tunnel: w366 -> [w397 w438]
              frame False {
                # "Otherwise, has CTD data, parse it and display temp, pressure, conductivity"
                n142 = property on="CTD Com Miss Count" class="DigNum (strict)"("Value"=0) -> ()  [unwired: 2 in, 2 out]
                n143 = property on="Winch Action Status" class="Enum (strict)"() -> ("Value"=w389:T1)  [unwired: 2 in, 2 out]
                n144 = Scan From String(format string="%d,%f,%f,%f", input string=w396, initial scan location=u32 0) -> (output 1=→"timestamp":u32, output 2=w390:dbl, output 3=→"Temperature":dbl, output 4=→"Conductivity":dbl)  [unwired: 5 in, 3 out]
                "Pressure" <- w390
                n145 = Greater?(x=w389, y=3) -> (0:w383:bool)
                n146 = call "Press2Depth.vi"("Pressure in dbars"=w390) -> ("Depth in meters"=w387:dbl)
                "Depth" <- w387
                n147 = property on="Drive by \nCTD Data" class="Bool (strict)"() -> ("Value"=w391:bool)  [unwired: 2 in, 2 out]
                n148 = property on="Max depth" class="DigNum (strict)"() -> ("Value"=w386:dbl)  [unwired: 2 in, 2 out]
                n149 = Greater?(x=w387, y="Maximum depth [m]") -> (0:w392:bool)
                n150 = And(x=w392, y=w391) -> (x .and. y?=w393:bool)
                n151 = Subtract(x=w397, y=w387) -> (x-y=→"Depth Derivative":dbl)
                n152 = stacked-sequence {
                  tunnel: [w405 _] -> _
                  tunnel: w387 -> [_ w423]
                  tunnel: "Maximum depth [m]" -> [_ w425]
                  tunnel: w393 -> [w405 _]
                  frame #0 {
                    n153 = case shown="True" w405 {
                      frame False {
                      }
                      frame True {
                        n154 = property on="isMaxPaySet" class="Bool (strict)"() -> ("Value"=w411:bool)  [unwired: 2 in, 2 out]
                        n155 = Not(x=w411) -> (.not. x?=w410:bool)
                        n156 = property on="Payout" class="Slide (strict)"() -> ("Value"=w413:dbl)  [unwired: 2 in, 2 out]
                        n157 = property on="Maximum payout [turns]" class="DigNum (strict)"() -> ("Value"=w412:dbl)  [unwired: 2 in, 2 out]
                        n158 = property on="Velocity Now" class="Knob (strict)"() -> ("Value"=w409:dbl)  [unwired: 2 in, 2 out]
                        n159 = Less?(x=w413, y=w412) -> (x < y?=w406:bool)
                        n160 = Greater Or Equal To 0?(x=w409) -> (x >= 0?=w407:bool)
                        n161 = And(x=w407, y=w406) -> (x .and. y?=w408:bool)
                        n162 = case shown="True" w410 {
                          selector: w410 -> [_ w414]
                          frame False {
                          }
                          frame True {
                            n163 = property on="isMaxPaySet" class="Bool (strict)"("Val(Sgnl)"=w414) -> ()  [unwired: 2 in, 2 out]
                            n164 = property on="Maximum payout [turns]" class="DigNum (strict)"() -> ("Value"=→"Old Max Payout":dbl)  [unwired: 2 in, 2 out]
                          }
                        }
                        n165 = case shown="True" w408 {
                          tunnel: w413 -> [_ w417]
                          frame False {
                          }
                          frame True {
                            n166 = Multiply(x=w417, y=0.8) -> (x*y=w416:dbl)
                            n167 = property on="Maximum payout [turns]" class="DigNum (strict)"("Val(Sgnl)"=w416) -> ()  [unwired: 2 in, 2 out]
                          }
                        }
                      }
                    }
                  }
                  frame #1 {
                    n168 = property on="Velocity Now" class="Knob (strict)"() -> ("Value"=w428:dbl)  [unwired: 2 in, 2 out]
                    n169 = property on="isMaxPaySet" class="Bool (strict)"() -> ("Value"=w421:bool)  [unwired: 2 in, 2 out]
                    n170 = Multiply(x=w425, y=0.8) -> (x*y=w424:dbl)
                    n171 = Greater?(x=w423, y=w424) -> (0:w422:bool)
                    n172 = Less Than 0?(x=w428) -> (x < 0?=w427:bool)
                    n173 = And(x=w427, y=w422) -> (x .and. y?=w420:bool)
                    n174 = And(x=w421, y=w420) -> (x .and. y?=w419:bool)
                    n175 = case shown="True" w419 {
                      selector: w419 -> [_ w430]
                      frame False {
                      }
                      frame True {
                        n176 = Not(x=w430) -> (.not. x?=w429:bool)
                        n177 = property on="isMaxPaySet" class="Bool (strict)"("Val(Sgnl)"=w429) -> ()  [unwired: 2 in, 2 out]
                        n178 = property on="Old Max Payout" class="DigNum (strict)"() -> ("Value"=w431:dbl)  [unwired: 2 in, 2 out]
                        n179 = property on="Maximum payout [turns]" class="DigNum (strict)"("Val(Sgnl)"=w431) -> ()  [unwired: 2 in, 2 out]
                      }
                    }
                  }
                }
                n180 = Less?(x=w386, y=w387) -> (x < y?=w385:bool)
                n181 = And(x=w383, y=w385) -> (x .and. y?=w384:bool)
                n182 = case shown="False" w383 {
                  frame False {
                    n183 = property on="Max depth" class="DigNum (strict)"("Value"=0.0) -> ()  [unwired: 2 in, 2 out]
                  }
                  frame True {
                  }
                }
                n184 = case shown="True" w384 {
                  tunnel: w387 -> [_ w434]
                  frame False {
                  }
                  frame True {
                    n185 = Get Date/Time In Seconds() -> (seconds since 1Jan1904=→"Time @ max":timestamp)
                    n186 = property on="Payout" class="Slide (strict)"() -> ("Value"=→"Max payout":dbl)  [unwired: 2 in, 2 out]
                    "Max depth" <- w434
                  }
                }
              }
              frame True {
                # "If CTD is emtpy string: increment CTD Miss count, and blink CTD bar"
                n187 = property on="CTD Com Miss Count" class="DigNum (strict)"() -> ("Value"=w439:dbl)  [unwired: 2 in, 2 out]
                n188 = Increment(x=w439) -> (x+1=w437:dbl)
                n189 = Greater?(x=w437, y=1) -> (0:w435:bool)
                n190 = property on="CTD data" class="Str"("Blinking"=w435) -> ()  [unwired: 2 in, 2 out]
                n191 = property on="Depth" class="Slide (strict)"("Blinking"=w435) -> ()  [unwired: 2 in, 2 out]
                n192 = property on="CTD Com Miss Count" class="DigNum (strict)"("Value"=w437) -> ()  [unwired: 2 in, 2 out]
                n193 = property on="Pressure" class="WFChart (strict)"("Blinking"=w435) -> ()  [unwired: 2 in, 2 out]
                n194 = property on="Depth Derivative" class="WFChart (strict)"("Blinking"=w435) -> ()  [unwired: 2 in, 2 out]
                n195 = property on="Conductivity" class="WFChart (strict)"("Blinking"=w435) -> ()  [unwired: 2 in, 2 out]
                n196 = property on="Temperature" class="WFChart (strict)"("Blinking"=w435) -> ()  [unwired: 2 in, 2 out]
              }
            }
            n197 = Bundle("Pressure"=w375, "Value"=w381) -> (→"Depth History":cluster{"Pressure ":dbl, "Value":dbl})  [unwired: 1 in]
          }
        }
      }
      frame #7 {
        # "Check for dead com links"
        n198 = stacked-sequence {
          seq-local: [w447 _] -> [_ w464]
          tunnel: w445 -> [w448 _]
          tunnel: [_ w464] -> w444
          tunnel: w443 -> [_ w465]
          tunnel: [_ w463] -> w442
          tunnel: w441 -> [w446 _]
          frame #0 {
            # "If winch miss count > 25, close connection and open again"
            n199 = property on="Winch Com Miss Count" class="DigNum (strict)"() -> ("Value"=w451:dbl)  [unwired: 2 in, 2 out]
            n200 = Greater?(x=w451, y=25) -> (0:w449:bool)
            n201 = case shown="True" w449 {
              tunnel: w448 -> [w452 w455]
              tunnel: [w452 w454] -> w447
              tunnel: w446 -> [_ w453]
              frame False {
              }
              frame True {
                n202 = stacked-sequence {
                  tunnel: w455 -> [w457 _ _]
                  tunnel: [_ _ w460] -> w454
                  tunnel: w453 -> [_ _ w458]
                  frame #0 {
                    n203 = TCP Close Connection(connection ID=w457) -> (error out=w456:errorcluster)  [unwired: 2 in, 1 out]
                    n204 = call <vilib>:"Clear Errors.vi"("error in (no error)"=w456) -> ()  [unwired: 5 in, 2 out]
                  }
                  frame #1 {
                    n205 = call "Time Delay"() -> ()  [unwired: 11 in, 1 out]
                  }
                  frame #2 {
                    n206 = TCP Open Connection(address=w458, remote port or service name=4050, timeout ms (60000)=1000) -> (connection ID=w460:refnum<k5>, error out=w459:errorcluster)  [unwired: 2 in]
                    n207 = call <vilib>:"Clear Errors.vi"("error in (no error)"=w459) -> ()  [unwired: 5 in, 2 out]
                  }
                }
              }
            }
          }
          frame #1 {
            # "If CTD miss count > 10, close connection and open again"
            n208 = property on="CTD Com Miss Count" class="DigNum (strict)"() -> ("Value"=w466:dbl)  [unwired: 2 in, 2 out]
            n209 = Greater?(x=w466, y=10) -> (0:w468:bool)
            n210 = case shown="True" w468 {
              tunnel: w465 -> [w469 w471]
              tunnel: [w469 w470] -> w463
              frame False {
              }
              frame True {
                n211 = stacked-sequence {
                  tunnel: w471 -> [w473 _ _ _]
                  tunnel: [_ _ _ w478] -> w470
                  frame #0 {
                    n212 = TCP Close Connection(connection ID=w473) -> (error out=w472:errorcluster)  [unwired: 2 in, 1 out]
                    n213 = call <vilib>:"Clear Errors.vi"("error in (no error)"=w472) -> ()  [unwired: 5 in, 2 out]
                  }
                  frame #1 {
                    n214 = call "Time Delay2"() -> ()  [unwired: 11 in, 1 out]
                  }
                  frame #2 {
                    n215 = property on="CTD Com Miss Count" class="DigNum (strict)"("Value"=0) -> ()  [unwired: 2 in, 2 out]
                  }
                  frame #3 {
                    n216 = property on="Port" class="DigNum (strict)"() -> ("Value"=w476:i32)  [unwired: 2 in, 2 out]
                    n217 = property on="CTD Data  IP Address" class="Str"() -> ("Value"=w477:string)  [unwired: 2 in, 2 out]
                    n218 = TCP Open Connection(address=w477, remote port or service name=w476, timeout ms (60000)=1000) -> (connection ID=w478:refnum<k5>, error out=w475:errorcluster)  [unwired: 2 in]
                    n219 = call <vilib>:"Clear Errors.vi"("error in (no error)"=w475) -> ()  [unwired: 5 in, 2 out]
                  }
                }
              }
            }
          }
        }
      }
      frame #8 {
        # "Check if the values set by the user \nand the values on the controls are the same"
        # "Image Capture of the Front Panel"
        n220 = property on="Enabled" class="Bool (strict)"() -> ("Value"=w480:bool)  [unwired: 2 in, 2 out]
        n221 = case shown="True" w480 {
          frame False {
          }
          frame True {
            n222 = property on="Min Payout" class="DigNum (strict)"() -> ("Value"=w520:dbl)  [unwired: 2 in, 2 out]
            n223 = property on="Minimum payout [turns]" class="DigNum (strict)"() -> ("Value"=w519:dbl)  [unwired: 2 in, 2 out]
            n224 = property on="Wire In Speed" class="DigNum (strict)"() -> ("Value"=w512:dbl)  [unwired: 2 in, 2 out]
            n225 = property on="Wire In Speed\n[turns/sec]" class="DigNum (strict)"() -> ("Value"=w511:dbl)  [unwired: 2 in, 2 out]
            n226 = property on="Maximum payout [turns]" class="DigNum (strict)"() -> ("Value"=w518:dbl)  [unwired: 2 in, 2 out]
            n227 = property on="Max Payout" class="DigNum (strict)"() -> ("Value"=w517:dbl)  [unwired: 2 in, 2 out]
            n228 = property on="Wire Out Speed\n[turns/sec]" class="DigNum (strict)"() -> ("Value"=w515:dbl)  [unwired: 2 in, 2 out]
            n229 = property on="Wire Out Speed" class="DigNum (strict)"() -> ("Value"=w514:dbl)  [unwired: 2 in, 2 out]
            n230 = Not Equal?(x=w519, y=w520) -> (x != y?=w521:bool)
            n231 = Not Equal?(x=w512, y=w511) -> (x != y?=w510:bool)
            n232 = Not Equal?(x=w518, y=w517) -> (x != y?=w516:bool)
            n233 = Not Equal?(x=w515, y=w514) -> (x != y?=w513:bool)
            n234 = property on="Minimum payout [turns]" class="DigNum (strict)"("Blinking"=w521) -> ()  [unwired: 2 in, 2 out]
            n235 = property on="Min Payout" class="DigNum (strict)"("Blinking"=w521) -> ()  [unwired: 2 in, 2 out]
            n236 = property on="Wire In Speed\n[turns/sec]" class="DigNum (strict)"("Blinking"=w510) -> ()  [unwired: 2 in, 2 out]
            n237 = property on="Maximum payout [turns]" class="DigNum (strict)"("Blinking"=w516) -> ()  [unwired: 2 in, 2 out]
            n238 = property on="Wire Out Speed\n[turns/sec]" class="DigNum (strict)"("Blinking"=w513) -> ()  [unwired: 2 in, 2 out]
            n239 = property on="Wire In Speed" class="DigNum (strict)"("Blinking"=w510) -> ()  [unwired: 2 in, 2 out]
            n240 = property on="Max Payout" class="DigNum (strict)"("Blinking"=w516) -> ()  [unwired: 2 in, 2 out]
            n241 = property on="Wire Out Speed" class="DigNum (strict)"("Blinking"=w513) -> ()  [unwired: 2 in, 2 out]
            n242 = property on="Stop decel out" class="DigNum (strict)"() -> ("Value"=w488:dbl)  [unwired: 2 in, 2 out]
            n243 = property on="Decel Stop Out" class="DigNum (strict)"() -> ("Value"=w487:dbl)  [unwired: 2 in, 2 out]
            n244 = property on="Final in Speed" class="DigNum (strict)"() -> ("Value"=w509:dbl)  [unwired: 2 in, 2 out]
            n245 = property on="Final In Speed\n[turns/sec]" class="DigNum (strict)"() -> ("Value"=w508:dbl)  [unwired: 2 in, 2 out]
            n246 = property on="Acc Out" class="DigNum (strict)"() -> ("Value"=w500:dbl)  [unwired: 2 in, 2 out]
            n247 = property on="Accel out" class="DigNum (strict)"() -> ("Value"=w499:dbl)  [unwired: 2 in, 2 out]
            n248 = property on="Acc In" class="DigNum (strict)"() -> ("Value"=w503:dbl)  [unwired: 2 in, 2 out]
            n249 = property on="Accel  in" class="DigNum (strict)"() -> ("Value"=w502:dbl)  [unwired: 2 in, 2 out]
            n250 = Not Equal?(x=w488, y=w487) -> (x != y?=w486:bool)
            n251 = Not Equal?(x=w509, y=w508) -> (x != y?=w507:bool)
            n252 = Not Equal?(x=w500, y=w499) -> (x != y?=w498:bool)
            n253 = Not Equal?(x=w503, y=w502) -> (x != y?=w501:bool)
            n254 = property on="Stop decel out" class="DigNum (strict)"("Blinking"=w486) -> ()  [unwired: 2 in, 2 out]
            n255 = property on="Decel Stop Out" class="DigNum (strict)"("Blinking"=w486) -> ()  [unwired: 2 in, 2 out]
            n256 = property on="Final in Speed" class="DigNum (strict)"("Blinking"=w507) -> ()  [unwired: 2 in, 2 out]
            n257 = property on="Final In Speed\n[turns/sec]" class="DigNum (strict)"("Blinking"=w507) -> ()  [unwired: 2 in, 2 out]
            n258 = property on="Accel out" class="DigNum (strict)"("Blinking"=w498) -> ()  [unwired: 2 in, 2 out]
            n259 = property on="Accel  in" class="DigNum (strict)"("Blinking"=w501) -> ()  [unwired: 2 in, 2 out]
            n260 = property on="Acc Out" class="DigNum (strict)"("Blinking"=w498) -> ()  [unwired: 2 in, 2 out]
            n261 = property on="Acc In" class="DigNum (strict)"("Blinking"=w501) -> ()  [unwired: 2 in, 2 out]
            n262 = property on="Decel Stop In" class="DigNum (strict)"() -> ("Value"=w491:dbl)  [unwired: 2 in, 2 out]
            n263 = property on="Stop decel in" class="DigNum (strict)"() -> ("Value"=w490:dbl)  [unwired: 2 in, 2 out]
            n264 = property on="Decel in" class="DigNum (strict)"() -> ("Value"=w497:dbl)  [unwired: 2 in, 2 out]
            n265 = property on="Decel In" class="DigNum (strict)"() -> ("Value"=w496:dbl)  [unwired: 2 in, 2 out]
            n266 = property on="Decel Out" class="DigNum (strict)"() -> ("Value"=w494:dbl)  [unwired: 2 in, 2 out]
            n267 = property on="Decel out" class="DigNum (strict)"() -> ("Value"=w493:dbl)  [unwired: 2 in, 2 out]
            n268 = property on="Slow Depth" class="DigNum (strict)"() -> ("Value"=w506:dbl)  [unwired: 2 in, 2 out]
            n269 = property on="Slow depth\n[turns]" class="DigNum (strict)"() -> ("Value"=w505:dbl)  [unwired: 2 in, 2 out]
            n270 = Not Equal?(x=w491, y=w490) -> (x != y?=w489:bool)
            n271 = Not Equal?(x=w497, y=w496) -> (x != y?=w495:bool)
            n272 = Not Equal?(x=w494, y=w493) -> (x != y?=w492:bool)
            n273 = Not Equal?(x=w506, y=w505) -> (x != y?=w504:bool)
            n274 = property on="Stop decel in" class="DigNum (strict)"("Blinking"=w489) -> ()  [unwired: 2 in, 2 out]
            n275 = property on="Decel in" class="DigNum (strict)"("Blinking"=w495) -> ()  [unwired: 2 in, 2 out]
            n276 = property on="Decel out" class="DigNum (strict)"("Blinking"=w492) -> ()  [unwired: 2 in, 2 out]
            n277 = property on="Decel Stop In" class="DigNum (strict)"("Blinking"=w489) -> ()  [unwired: 2 in, 2 out]
            n278 = property on="Decel In" class="DigNum (strict)"("Blinking"=w495) -> ()  [unwired: 2 in, 2 out]
            n279 = property on="Decel Out" class="DigNum (strict)"("Blinking"=w492) -> ()  [unwired: 2 in, 2 out]
            n280 = property on="Slow depth\n[turns]" class="DigNum (strict)"("Blinking"=w504) -> ()  [unwired: 2 in, 2 out]
            n281 = property on="Slow Depth" class="DigNum (strict)"("Blinking"=w504) -> ()  [unwired: 2 in, 2 out]
          }
        }
        n282 = Get Date/Time In Seconds() -> (seconds since 1Jan1904=w485:timestamp)
        n283 = Format Date/Time String(seconds (now)=w485) -> (date/time string=w484:string)  [unwired: 2 in]
        n284 = Concatenate Strings("Updated: ", w484) -> (→"Last update string":string)
        n285 = case shown="True" "Screen Capture" {
          frame False {
            n286 = property on="Path of Image Capture" class="Path"("DisabledEnum"=2) -> ()  [unwired: 2 in, 2 out]
          }
          frame True {
            n287 = property on="Path of Image Capture" class="Path"("DisabledEnum"=0) -> ()  [unwired: 2 in, 2 out]
            n288 = feedback #1() -> (w523:errorcluster)  [unwired: 1 in]
            n289 = call <vilib>:"Check if File or Folder Exists.vi"("error in (no error)"=w523, "path"="Path of Image Capture") -> ("error out"=w525:errorcluster, "file or folder exists?"=w527:bool, "dup path"=w528:path)  [unwired: 7 in]
            n290 = case shown="True" w527 {
              tunnel: w528 -> [w536 w538]
              tunnel: w525 -> [w531 _]
              tunnel: [w530 w537] -> w524
              frame False {
                n291 = Open/Create/Replace File(file path (use dialog)=w536, error in=w531, operation (0:open)=4, access (0:read/write)=0) -> (refnum out=w532:refnum<file>, error out=w533:errorcluster)  [unwired: 2 in, 1 out]
                n292 = Close File(refnum=w532, error in=w533) -> (error out=w530:errorcluster)  [unwired: 1 out]
              }
              frame True {
                # "Close VI ref"
                # "24 bit image depth"
                # "Open VI Reference Function"
                # "Current VI's Path"
                # "Save an image capture of the Fron Panel"
                n293 = Current VI's Path() -> (path=w545:path)
                n294 = Open VI Reference(vi path=w545) -> (vi reference=w542:refnum<vi>, error out=w544:errorcluster)  [unwired: 5 in]
                n295 = invoke class="VI" method="FP.Get Image"(reference=w542, error in=w544, "image depth"=24) -> (reference out=w540:refnum<vi>, error out=w541:errorcluster, "image data"=w543:T5)  [unwired: 3 in, 3 out]
                n296 = Close Reference(reference=w540) -> ()  [unwired: 1 in, 1 out]
                n297 = call <vilib>:"Write PNG File.vi"("error in (no error)"=w541, "image data"=w543, "path to PNG file"=w538) -> ("error out"=w537:errorcluster)  [unwired: 7 in, 1 out]
              }
            }
            n298 = feedback-in #1(w524) -> ()
          }
        }
      }
    }
  }
  n299 = Strip Path(path=w9) -> (stripped path=w8:path)  [unwired: 1 out]
  n300 = Strip Path(path=w8) -> (stripped path=w7:path)  [unwired: 1 out]
  n301 = Build Path(base path=w7, name or relative path="Sites") -> (appended path=w5:path)
  n302 = Build Path(base path=w5, name or relative path="FCTD_WINCH") -> (appended path=w3:path)
  n303 = Build Path(base path=w3, name or relative path="LabView.png") -> (appended path=w1:path)
  n304 = property on="Path of Image Capture" class="Path"("Value"=w1) -> ()  [unwired: 2 in, 2 out]
  n305 = TCP Close Connection(connection ID=w18, error in (no error)=w51) -> (error out=w20:errorcluster)  [unwired: 1 in, 1 out]
  n306 = TCP Close Connection(connection ID=w27, error in (no error)=w25) -> (error out=w29:errorcluster)  [unwired: 1 in, 1 out]
  n307 = call <vilib>:"Simple Error Handler.vi"("error in (no error)"=w20) -> ()  [unwired: 4 in, 5 out]
  n308 = call <vilib>:"Simple Error Handler.vi"("error in (no error)"=w29) -> ()  [unwired: 4 in, 5 out]
  "CTD Com Miss Count" <- w19
  "Winch Com Miss Count" <- w19
  "isMaxPaySet" <- FALSE
  "RL Status Received" <- FALSE
